vi "EMG_Signal_Mean_Amplitude_Computation.vi"(6 "Greater than first threshold?":bool, 7 "EMG signal (V)":dbl, 9 "Greater than second threshold?":bool, 10 "Contracted?":bool, 11 "Harder contracted?":bool) -> (2 "Mean signal amplitude (V)":dbl)   [LabVIEW 2015]
uses:
  <vilib>/ptbypt/NI_PtbyPt.lvlib
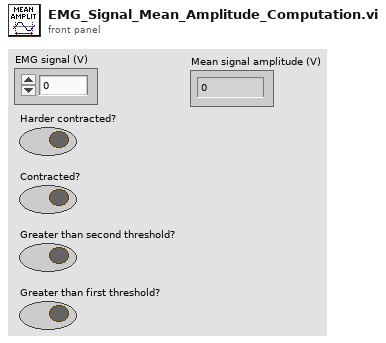
[diagram p1: front panel]
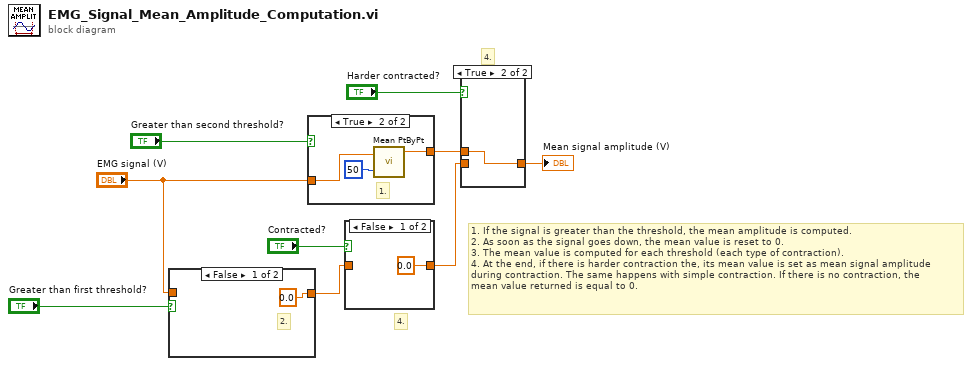
[diagram p0: block diagram]
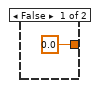
[diagram p4: hidden frame]
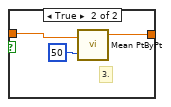
[diagram p5: hidden frame]
diagram:
  # "4."
  # "4."
  # "1. If the signal is greater than the threshold, the mean amplitude is computed.\n2. As soon as the signal goes down, the mean value is reset to 0.\n3. The mean value is computed for each threshold (each type of contraction).\n4. At the end, if there is harder contraction the, its mean value is set as mean signal amplitude\nduring contraction. The same happens with simple contraction. If there is no contraction, the\nmean value returned is equal to 0."
  n1 = case shown="False" "Greater than first threshold?" {
    tunnel: "EMG signal (V)" -> [_ w13]
    tunnel: [0.0 ("mean") w12] -> w8
    frame False {
      # "2."
    }
    frame True {
      # "3."
      n2 = call <vilib>:"Mean PtByPt.vi"("x"=w13, "sample length"=50) -> ("mean"=w12:dbl)  [unwired: 2 in, 1 out]
    }
  }
  n3 = case shown="True" "Greater than second threshold?" {
    tunnel: "EMG signal (V)" -> [_ w17]
    tunnel: [0.0 ("mean") w16] -> w6
    frame False {
    }
    frame True {
      # "1."
      n4 = call <vilib>:"Mean PtByPt.vi"("x"=w17, "sample length"=50) -> ("mean"=w16:dbl)  [unwired: 2 in, 1 out]
    }
  }
  n5 = case shown="False" "Contracted?" {
    tunnel: [0.0 ("mean") w19] -> w9
    tunnel: w8 -> [_ w19]
    frame False {
    }
    frame True {
    }
  }
  n6 = case shown="True" "Harder contracted?" {
    tunnel: [w20 w21] -> w1
    tunnel: w6 -> [_ w21]
    tunnel: w9 -> [w20 _]
    frame False {
    }
    frame True {
    }
  }
  "Mean signal amplitude (V)" <- w1
